vi "HIOKI PW3390 Conf Aout.vi"(0 "VISA Resource":refnum<visa-resource-name>, 1 "Frequency f.s. (3: 5kHz)":enum16{"100Hz", "500Hz", "1kHz", "5kHz"}(ring)=enum."5kHz", 2 "Integrate f.s. (2: 1)":T3(ring)=enum."1", 3 "Item":T2(array[cluster])=[{"Item"=enum."Urms", "Ch(0:Ch1)"=enum."1"}, {"Item"=enum."Urms", "Ch(0:Ch1)"=enum."1"}, {"Item"=enum."Urms", "Ch(0:Ch1)"=enum."1"}, {"Item"=enum."Urms", "Ch(0:Ch1)"=enum."1"}, {"Item"=enum."Urms", "Ch(0:Ch1)"=enum."1"}, {"Item"=enum."Urms", "Ch(0:Ch1)"=enum."1"}, {"Item"=enum."Urms", "Ch(0:Ch1)"=enum."1"}, {"Item"=enum."Urms", "Ch(0:Ch1)"=enum."1"}, {"Item"=enum."Urms", "Ch(0:Ch1)"=enum."1"}, {"Item"=enum."Urms", "Ch(0:Ch1)"=enum."1"}, {"Item"=enum."Urms", "Ch(0:Ch1)"=enum."1"}, {"Item"=enum."Urms", "Ch(0:Ch1)"=enum."1"}, {"Item"=enum."Urms", "Ch(0:Ch1)"=enum."1"}, {"Item"=enum."Urms", "Ch(0:Ch1)"=enum."1"}, {"Item"=enum."Urms", "Ch(0:Ch1)"=enum."1"}, {"Item"=enum."Urms", "Ch(0:Ch1)"=enum."1"}], 4 "Wave Output (T: ON)":bool=TRUE, 5 "error in (no error)":errorcluster, 6 "Set/Query (F: Set)":bool, 7 "Output Range (1: 2V f.s.)":enum16{"1", "2"}(ring)=enum."2", 9 "OPC query (T: ON)":bool=TRUE, 11 "Error Out (F: Off)":bool) -> (13 "Output Range out":enum16{"1", "2"}(ring)=3, 14 "VISA Resource out":refnum<visa-resource-name>, 15 "Frequency f.s. out":enum16{"100Hz", "500Hz", "1kHz", "5kHz"}(ring)=enum."5kHz", 16 "Integrate f.s. out":T3(ring)=enum."1", 17 "Item out":T1(array[cluster])=[{"Item"=enum."Urms", "Numerator"=enum."1"}, {"Item"=enum."Urms", "Numerator"=enum."1"}, {"Item"=enum."Urms", "Numerator"=enum."1"}, {"Item"=enum."Urms", "Numerator"=enum."1"}, {"Item"=enum."Urms", "Numerator"=enum."1"}, {"Item"=enum."Urms", "Numerator"=enum."1"}, {"Item"=enum."Urms", "Numerator"=enum."1"}, {"Item"=enum."Urms", "Numerator"=enum."1"}, {"Item"=enum."Urms", "Numerator"=enum."1"}, {"Item"=enum."Urms", "Numerator"=enum."1"}, {"Item"=enum."Urms", "Numerator"=enum."1"}, {"Item"=enum."Urms", "Numerator"=enum."1"}, {"Item"=enum."Urms", "Numerator"=enum."1"}, {"Item"=enum."Urms", "Numerator"=enum."1"}, {"Item"=enum."Urms", "Numerator"=enum."1"}, {"Item"=enum."Urms", "Numerator"=enum."1"}], 18 "Wave Output out":bool=TRUE, 19 "error out":errorcluster)   [LabVIEW 2009]
doc: "Sets and reads the functions related to D/A Output.\n\nSet/Query\n Set: Send the setting commands for the device.\n Query: Query the setting of the device.\n\nFrequency f.s.\n Sets the frequency full scale and the motor's maximum frequency.\n\nIntegrate f.s.\n Sets the Integration full scale coefficients.\n\nItem\n Sets the D/A Output Items (Item, CH).\n Specifies the output items between 1 and 16.\n\nWave Output\n Sets the ON/OFF of the waveform output.\n\nOutput Range\n Sets the full scale of the waveform output."
panel:
  # "Item(1: Urms)"
  # "Ch"
  # "Ch(0:Ch1)"
  # "Item"
  # "AOut1"
  # "AOut1"
  # "AOut2"
  # "AOut2"
  # "AOut3"
  # "AOut3"
  # "AOut4"
  # "AOut4"
  # "AOut5"
  # "AOut5"
  # "AOut6"
  # "AOut6"
  # "AOut7"
  # "AOut7"
  # "AOut8"
  # "AOut8"
  # "AOut9"
  # "AOut9"
  # "AOut10"
  # "AOut10"
  # "AOut11"
  # "AOut11"
  # "AOut12"
  # "AOut12"
  # "AOut13"
  # "AOut13"
  # "AOut14"
  # "AOut14"
  # "AOut15"
  # "AOut15"
  # "AOut16"
  # "AOut16"
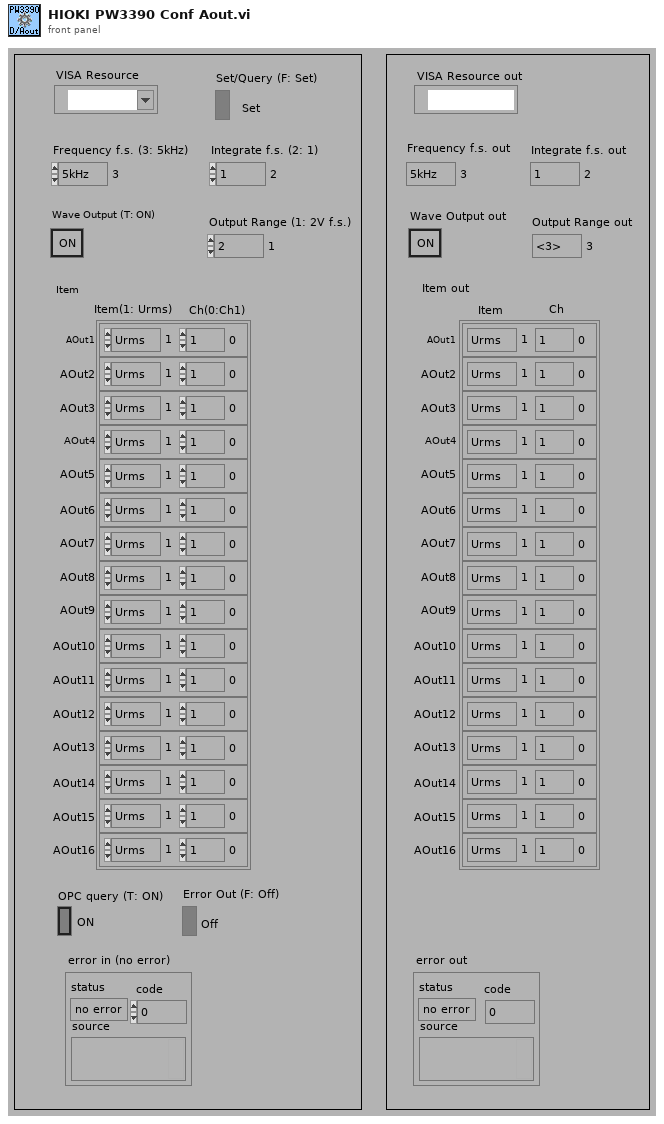
[diagram p1: front panel]
types:
  T1 = cluster{"Item":enum16{"OFF", "Urms", "Umn", "Uac", "Udc", "Ufnd", "Upk+", "Upk-", "Uthd", "Urf", "Uunb", "Irms", "Imn", "Iac", "Idc", "Ifnd", "Ipk+", "Ipk-", "Ithd", "Irf", "Iunb", "P", "S", "Q", "PF", "DEG U", "DEG I", "DEG P", "f", "EFFI", "LOSS", "IH+", "IH-", "IH", "WP+", "WP-", "WP", "CH A", "CH B", "Pm", "Slip"}, "Numerator":enum16{"1", "2", "3", "4", "12", "34", "123"}}[]
  T2 = cluster{"Item":enum16{"OFF", "Urms", "Umn", "Uac", "Udc", "Ufnd", "Upk+", "Upk-", "Uthd", "Urf", "Uunb", "Irms", "Imn", "Iac", "Idc", "Ifnd", "Ipk+", "Ipk-", "Ithd", "Irf", "Iunb", "P", "S", "Q", "PF", "DEG U", "DEG I", "DEG P", "f", "EFFI", "LOSS", "IH+", "IH-", "IH", "WP+", "WP-", "WP", "CH A", "CH B", "Pm", "Slip"}, "Ch(0:Ch1)":enum16{"1", "2", "3", "4", "12", "34", "123"}}[]
  T3 = enum16{"1/10", "1/2", "1", "5", "10", "50", "100", "500", "1000", "5000", "10000"}
  T4 = enum16{"OFF", "Urms", "Umn", "Uac", "Udc", "Ufnd", "Upk+", "Upk-", "Uthd", "Urf", "Uunb", "Irms", "Imn", "Iac", "Idc", "Ifnd", "Ipk+", "Ipk-", "Ithd", "Irf", "Iunb", "P", "S", "Q", "PF", "DEG U", "DEG I", "DEG P", "f", "EFFI", "LOSS", "IH+", "IH-", "IH", "WP+", "WP-", "WP", "CH A", "CH B", "Pm", "Slip"}
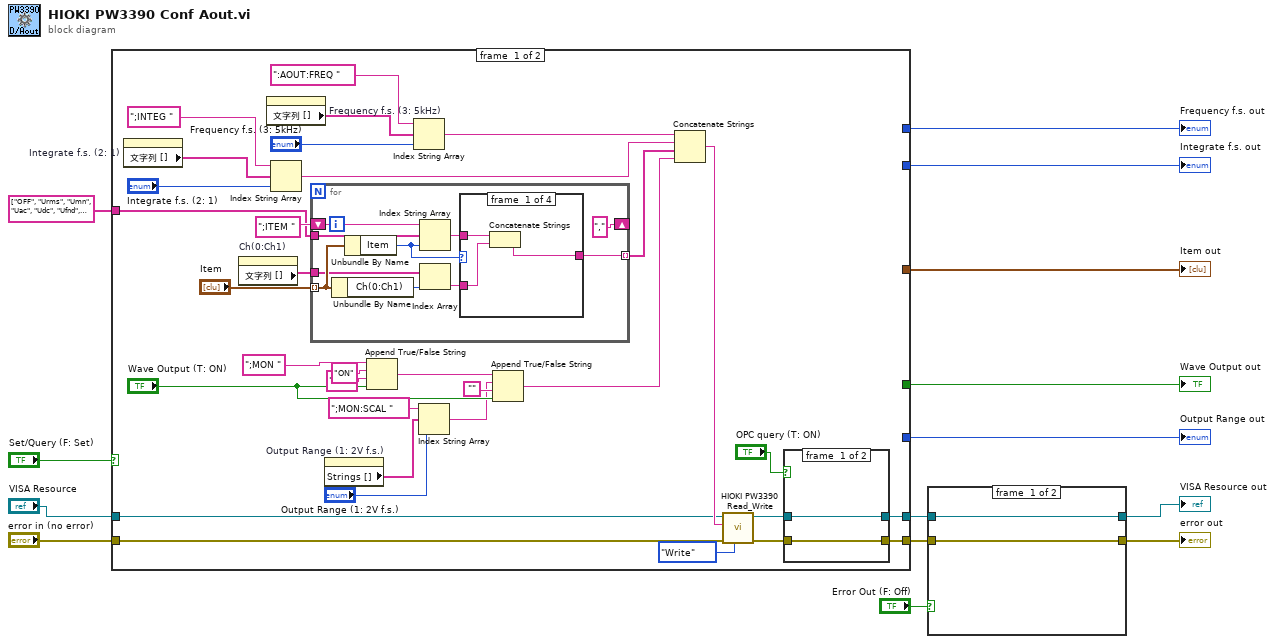
[diagram p0: block diagram]
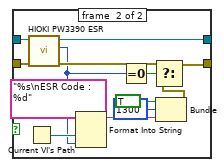
[diagram p2: hidden frame]
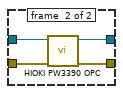
[diagram p3: hidden frame]
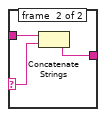
[diagram p5: hidden frame]
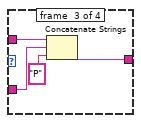
[diagram p6: hidden frame]
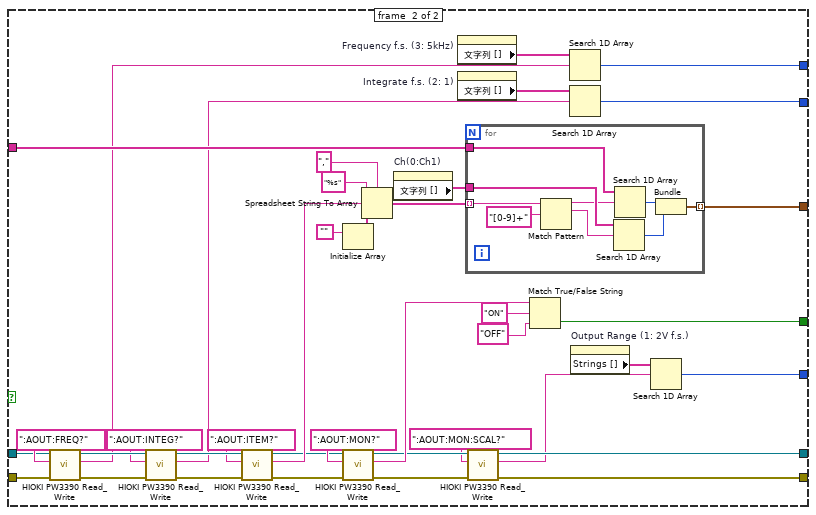
[diagram p8: hidden frame]
diagram:
  n1 = case shown="FALSE" "Set/Query (F: Set)" {
    tunnel: "error in (no error)" -> [w40 w117]
    tunnel: [w23 w83] -> w7
    tunnel: [w24 w84] -> w6
    tunnel: [_ w94] -> w12
    tunnel: [_ w87] -> w11
    tunnel: [_ w103] -> w10
    tunnel: [_ w95] -> w9
    tunnel: string[] ["OFF", "Urms", "Umn", "Uac", "Udc", "Ufnd", "PUpk", "MUpk", "Uthd", "Urf", "Uunb", "Irms", "Imn", "Iac", "Idc", "Ifnd", "PIpk", "MIpk", "Ithd", "Irf", "Iunb", "P", "S", "Q", "PF", "HU", "HI", "DEG", "FREQ", "Eff", "Loss", "PIH", "MIH", "IH", "PWP", "MWP", "WP", "ExtA", "ExtB", "Pm", "Slip", ""] ("Strings []") -> [w32 w93]
    tunnel: "VISA Resource" -> [w28 w88]
    tunnel: [_ w79] -> w1
    frame #0 {
      n2 = property on="Integrate f.s. (2: 1)" class="Enum (strict)"() -> ("文字列 []"=w43:string[])  [unwired: 2 in, 2 out]
      n3 = property on="Ch(0:Ch1)" class="Enum (strict)"() -> ("文字列 []"=w31:string[])  [unwired: 2 in, 2 out]
      n4 = property on="Frequency f.s. (3: 5kHz)" class="Enum (strict)"() -> ("文字列 []"=w46:string[])  [unwired: 2 in, 2 out]
      n5 = Index String Array(1:"Integrate f.s. (2: 1)", 2:w43, 3:";INTEG ") -> (0:w36:string)
      n6 = for {
        shift-right: [","] -> _
        shift-left: ";ITEM " -> [w63]
        tunnel: [w55] -> w29 mode=indexing
        tunnel: "Item" -> [w61] mode=indexing
        tunnel: w32 -> [w60]
        tunnel: w31 -> [w59]
        n7 = Unbundle By Name(w61) -> ("Ch(0:Ch1)"=w54:enum16{"1", "2", "3", "4", "12", "34", "123"})
        n8 = Unbundle By Name(w61) -> ("Item"=w56:T4)
        n9 = Index String Array(1:w56, 2:w60, 3:w63) -> (0:w58:string)
        n10 = Index Array(array=w59, index=w54) -> (element=w57:string)
        n11 = case shown="\"OFF\", \"CH A\".." w56 {
          tunnel: w58 -> [w66 w69 w77 w78]
          tunnel: w57 -> [w65 w67 w76 _]
          tunnel: [w64 w68 w75 w78] -> w55
          frame #0 {
            n12 = Concatenate Strings(w66, w65) -> (w64:string)
          }
          frame #1 {
            n13 = case shown="デフォルト" w67 {
              selector: w67 -> [_ w71]
              tunnel: w69 -> [w70 w73]
              tunnel: [w70 w72] -> w68
              frame #0 {
              }
              frame #1 {
                n14 = Concatenate Strings(w73, w71) -> (w72:string)
              }
            }
          }
          frame #2 {
            n15 = Concatenate Strings(w77, w76, "P" ("文字列")) -> (w75:string)
          }
          frame #3 {
          }
        }
      }
      n16 = property on="Output Range (1: 2V f.s.)" class="Enum （指定）"() -> ("Strings []"=w16:string[])  [unwired: 2 in, 2 out]
      n17 = Append True/False String(1:"Wave Output (T: ON)", 2:"OFF", 3:"ON", 4:";MON ") -> (0:w19:string)
      n18 = Index String Array(1:"Frequency f.s. (3: 5kHz)", 2:w46, 3:":AOUT:FREQ ") -> (0:w35:string)
      n19 = Index String Array(1:"Output Range (1: 2V f.s.)", 2:w16, 3:";MON:SCAL ") -> (0:w18:string)
      n20 = Append True/False String(1:"Wave Output (T: ON)", 2:"", 3:w18, 4:w19) -> (0:w22:string)
      n21 = Concatenate Strings(w35, w36, w29, w22) -> (w34:string)
      n22 = call <instrlib>:"HIOKI PW3390 Read_Write.vi"("Read/Write"=enum16{"Read", "Write"}."Write", "error in (no error)"=w40, "data in"=w34, "VISA Resource"=w28) -> ("error out"=w25:errorcluster, "VISA Resource out"=w26:refnum<visa-resource-name>)  [unwired: 5 in, 1 out]
      n23 = case shown="TRUE" "OPC query (T: ON)" {
        tunnel: [w49 w53] -> w24
        tunnel: [w48 w52] -> w23
        tunnel: w26 -> [w49 w51]
        tunnel: w25 -> [w48 w50]
        frame #0 {
        }
        frame #1 {
          n24 = call <instrlib>:"HIOKI PW3390 OPC.vi"("error in (no error)"=w50, "VISA Resource"=w51) -> ("error out"=w52:errorcluster, "VISA Resource out"=w53:refnum<visa-resource-name>)  [unwired: 7 in, 1 out]
        }
      }
    }
    frame #1 {
      n25 = call <instrlib>:"HIOKI PW3390 Read_Write.vi"("error in (no error)"=w117, "data in"=":AOUT:FREQ?", "VISA Resource"=w88) -> ("error out"=w113:errorcluster, "data out"=w91:string, "VISA Resource out"=w116:refnum<visa-resource-name>)  [unwired: 6 in]
      n26 = call <instrlib>:"HIOKI PW3390 Read_Write.vi"("error in (no error)"=w113, "data in"=":AOUT:INTEG?", "VISA Resource"=w116) -> ("error out"=w114:errorcluster, "data out"=w90:string, "VISA Resource out"=w115:refnum<visa-resource-name>)  [unwired: 6 in]
      n27 = call <instrlib>:"HIOKI PW3390 Read_Write.vi"("error in (no error)"=w114, "data in"=":AOUT:ITEM?", "VISA Resource"=w115) -> ("error out"=w99:errorcluster, "data out"=w104:string, "VISA Resource out"=w100:refnum<visa-resource-name>)  [unwired: 6 in]
      n28 = Initialize Array("") -> (w108:string[])  [unwired: 1 in]
      n29 = call <instrlib>:"HIOKI PW3390 Read_Write.vi"("error in (no error)"=w99, "data in"=":AOUT:MON?", "VISA Resource"=w100) -> ("error out"=w85:errorcluster, "data out"=w98:string, "VISA Resource out"=w86:refnum<visa-resource-name>)  [unwired: 6 in]
      n30 = Spreadsheet String To Array(delimiter (Tab)=",", format string="%s", spreadsheet string=w104, array type (2D Dbl)=w108) -> (array=w109:string[])
      n31 = property on="Ch(0:Ch1)" class="Enum (strict)"() -> ("文字列 []"=w102:string[])  [unwired: 2 in, 2 out]
      n32 = property on="Frequency f.s. (3: 5kHz)" class="Enum (strict)"() -> ("文字列 []"=w92:string[])  [unwired: 2 in, 2 out]
      n33 = property on="Integrate f.s. (2: 1)" class="Enum (strict)"() -> ("文字列 []"=w89:string[])  [unwired: 2 in, 2 out]
      n34 = for {
        tunnel: w109 -> [w120] mode=indexing
        tunnel: [w125] -> w103 mode=indexing
        tunnel: w93 -> [w123]
        tunnel: w102 -> [w122]
        n35 = Match Pattern(string=w120, regular expression="[0-9]+" ("正規表現")) -> (before substring=w118:string, match substring=w119:string)  [unwired: 1 in, 2 out]
        n36 = Search 1D Array(1D array=w122, element=w119) -> (index of element=w124:i32)  [unwired: 1 in]
        n37 = Search 1D Array(1D array=w123, element=w118) -> (index of element=w126:i32)  [unwired: 1 in]
        n38 = Bundle("要素の指標"=w126, "要素の指標"=w124) -> (w125:cluster{"要素の指標":i32, "要素の指標":i32})  [unwired: 1 in]
      }
      n39 = call <instrlib>:"HIOKI PW3390 Read_Write.vi"("error in (no error)"=w85, "data in"=":AOUT:MON:SCAL?", "VISA Resource"=w86) -> ("error out"=w83:errorcluster, "data out"=w81:string, "VISA Resource out"=w84:refnum<visa-resource-name>)  [unwired: 6 in]
      n40 = Match True/False String(2:"OFF" ("true文字列"), 3:"ON" ("true文字列"), 4:w98) -> (0:w95:bool)  [unwired: 1 out]
      n41 = Search 1D Array(1D array=w92, element=w91) -> (index of element=w94:i32)  [unwired: 1 in]
      n42 = Search 1D Array(1D array=w89, element=w90) -> (index of element=w87:i32)  [unwired: 1 in]
      n43 = property on="Output Range (1: 2V f.s.)" class="Enum （指定）"() -> ("Strings []"=w80:string[])  [unwired: 2 in, 2 out]
      n44 = Search 1D Array(1D array=w80, element=w81) -> (index of element=w79:i32)  [unwired: 1 in]
    }
  }
  "Integrate f.s. out" <- w11
  "Frequency f.s. out" <- w12
  "Item out" <- w10
  "Wave Output out" <- w9
  "Output Range out" <- w1
  n45 = case shown="TRUE" "Error Out (F: Off)" {
    tunnel: w6 -> [w127 w141]
    tunnel: w7 -> [w128 w140]
    tunnel: [w128 w131] -> w5
    tunnel: [w127 w129] -> w2
    frame #0 {
    }
    frame #1 {
      n46 = Current VI's Path() -> (path=w138:path)
      n47 = call <instrlib>:"HIOKI PW3390 ESR.vi"("error in (no error)"=w140, "VISA Resource"=w141) -> ("error out"=w132:errorcluster, "Output Value"=w130:u8, "VISA Resource out"=w129:refnum<visa-resource-name>)  [unwired: 6 in, 1 out]
      n48 = Format Into String(format string="%s\nESR Code : %d", w138, w130) -> (resulting string=w134:string)  [unwired: 2 in, 1 out]
      n49 = Equal To 0?(x=w130) -> (x = 0?=w139:bool)
      n50 = Bundle("status"=TRUE, "code"=1300, w134) -> (w133:cluster{"status":bool, "code":i32, string})  [unwired: 1 in]
      n51 = Select(t=w132, s=w139, f=w133) -> (s? t:f=w131:errorcluster)
    }
  }
  "error out" <- w5
  "VISA Resource out" <- w2
